vi "Warning Message by Frank.vi"(8 "Contiuous":bool, 9 "cancel":bool, 10 "ok?":bool, 11 "Arm Flag":bool) -> (1 "super cancel":bool=TRUE, 2 "super ok":bool=TRUE, 3 "Warning Message":string="NO WARNING!\n:)")   [LabVIEW 2018]
panel:
  out "Continuous?":bool
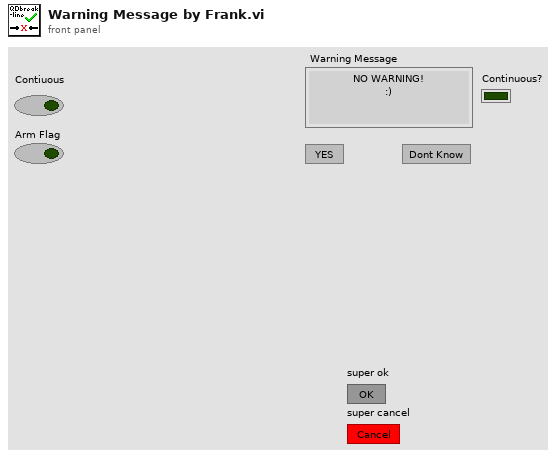
[diagram p1: front panel]
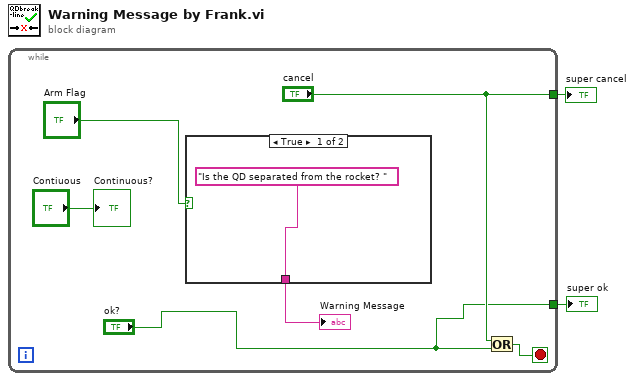
[diagram p0: block diagram]
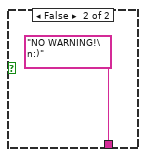
[diagram p2: hidden frame]
diagram:
  n1 = while {
    tunnel: ["cancel"] -> w2
    tunnel: ["ok?"] -> w1
    stop <- w6 stop-if-true
    n2 = case shown="True" "Arm Flag" {
      tunnel: ["Is the QD separated from the rocket? " "NO WARNING!\n:)"] -> w8
      frame True {
      }
      frame False {
      }
    }
    "Warning Message" <- w8
    n3 = Or(x="cancel", y="ok?") -> (x .or. y?=w6:bool)
    "Continuous?" <- "Contiuous"
  }
  "super cancel" <- w2
  "super ok" <- w1
